vi "suma de numeros divisibles pro 3.vi"() -> ()   [LabVIEW 2020]
panel:
  out "Numeric 2":dbl
  out "Numeric":dbl
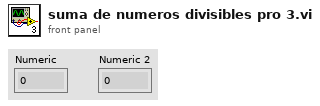
[diagram p1: front panel]
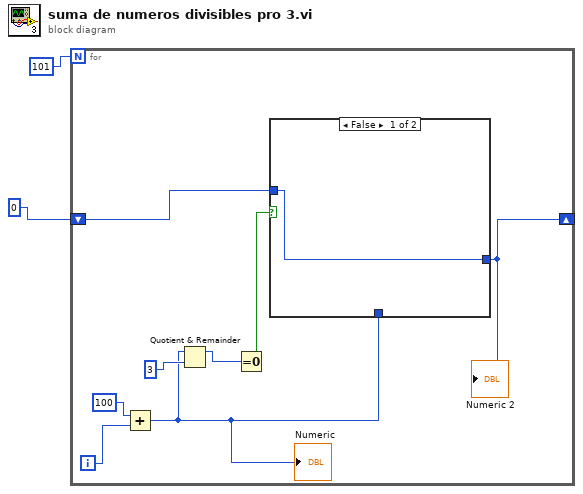
[diagram p0: block diagram]
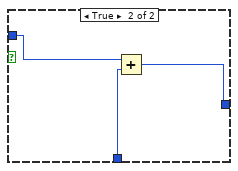
[diagram p2: hidden frame]
diagram:
  n1 = for {
    N: 101 -> [_]
    shift-right: [w3] -> _
    shift-left: 0 -> [w5]
    i -> [w10]
    n2 = Add(x=100, y=w10) -> (x+y=w4:i32)
    "Numeric" <- w4
    n3 = Quotient & Remainder(x=w4, y=3) -> (x-y*floor(x/y)=w8:i32)  [unwired: 1 out]
    n4 = Equal To 0?(x=w8) -> (x = 0?=w6:bool)
    n5 = case shown="False" w6 {
      tunnel: w4 -> [_ w14]
      tunnel: w5 -> [w11 w13]
      tunnel: [w11 w12] -> w3
      frame False {
      }
      frame True {
        n6 = Add(x=w13, y=w14) -> (x+y=w12:i32)
      }
    }
    "Numeric 2" <- w3
  }
